vi "4155C Transfer v2.0.vi"(0 "VISA resource name in":refnum<visa-resource-name>="GPIB0::14::INSTR", 1 "Source/Common":u32(ring) items=["SMU1  ", "SMU2  ", "SMU3  ", "SMU4  ", "SMU5  ", "SMU6  "], 2 "Gate":T5={"Gate Start"=0.0, "Gate Stop"=2.0, "Gate Step (linear only)"=1.0, "Gate Compliance"=0.0001, "Gate PComp"=0.0, "Range mode"=0, "Range"=6} {"Range" max=11 scale=0.0..11.0; "Range mode" items=["Auto", "Limited", "Fixed"]; "Gate PComp" min=0.0 max=2.0 format="%^.2e"; "Gate Compliance" min=0.0 max=0.1 format="%^.2e"; "Gate Step (linear only)" min=-100.0 max=100.0 format="%^.4e"; "Gate Stop" min=-100.0 max=100.0 format="%^.4e"; "Gate Start" min=-100.0 max=100.0 format="%^.4e"}, 3 "Drain":T6={"Drain Start"=0.0, "Drain Stop"=2.0, "Drain Compliance"=0.0001, "Drain Step"=1.0, "Drain PComp"=0.0, "Range mode"=0, "Range"=6} {"Range" max=11 scale=0.0..11.0; "Range mode" items=["Auto", "Limited", "Fixed"]; "Drain PComp" min=0.0 max=2.0 format="%^.2e"; "Drain Step" min=-100.0 max=100.0 format="%^.4e"; "Drain Compliance" min=0.0 max=0.1 format="%^.2e"; "Drain Stop" min=-100.0 max=100.0 format="%^.4e"; "Drain Start" min=-100.0 max=100.0 format="%^.4e"}, 4 "Drain":u32(ring)=1 items=["SMU1  ", "SMU2  ", "SMU3  ", "SMU4  ", "SMU5  ", "SMU6  "], 5 "Timings":T4={"integration time"=0, "Short/Long integration time"=0.00064, "hold time (sec)"=0.0, "delay time (sec)"=0.0, "Step Time (0 disables)"=0.0, "sweep method"=0, "Pulse period"=0.005, "Base voltage"=0.0, "Pulse width"=0.0005} {"Pulse width" min=0.0005 max=0.1 step=0.0001 format="%.4f"; "Base voltage" min=-100.0 max=100.0 format="%^.4e"; "Pulse period" min=0.005 max=1.0 step=0.0001 format="%.4f"; "sweep method" items=["Continuous", "Pulsed"]; "Step Time (0 disables)" min=0.0 format="%.2f"; "delay time (sec)" min=0.0 format="%.4f"; "hold time (sec)" min=0.0 format="%.4f"; "Short/Long integration time" min=0.0 format="%^.0e"; "integration time" scale=0.0..2.0}, 6 "error in (no error)":errorcluster, 7 "Probe 4":cluster{"on/off":bool, "Voltage":dbl} {"Voltage" min=-100.0 max=100.0 format="%.2f"}, 8 "Gate":u32(ring)=2 items=["SMU1  ", "SMU2  ", "SMU3  ", "SMU4  ", "SMU5  ", "SMU6  "], 9 "Probe 4":u32(ring)=3 items=["SMU1  ", "SMU2  ", "SMU3  ", "SMU4  ", "SMU5  ", "SMU6  "], 10 "sweep mode":u16(ring) items=["Single", "Double"], 12 "Panel Controls":T3={"Emergency Stop"=refnum, "TransGraph Max"=1e-05, "Text/Graph (text=false)"=FALSE, "TransGraph Min"=1e-11} {"TransGraph Min" format="%.2e"; "TransGraph Max" format="%.2e"}, 13 "Standby":T1) -> (16 "VG":dbl[](array[numeric]) format="%.2f", 17 "Outparams":T2={"V2 Start"=0.0, "V2 Step"=0.0, "Number of points"=1} {"V2 Step" format="%.2f"; "V2 Start" format="%^.4e"}, 20 "VISA Resource Name out":refnum<visa-resource-name>, 22 "IS":dbl[](array[numeric]) format="%.2f", 23 "ID":dbl[](array[numeric]) format="%.2f", 25 "IG":dbl[](array[numeric]) format="%.2f", 26 "error out":errorcluster, 27 "Probe 4":dbl[](array[numeric]) format="%.2f")   [LabVIEW 2016]
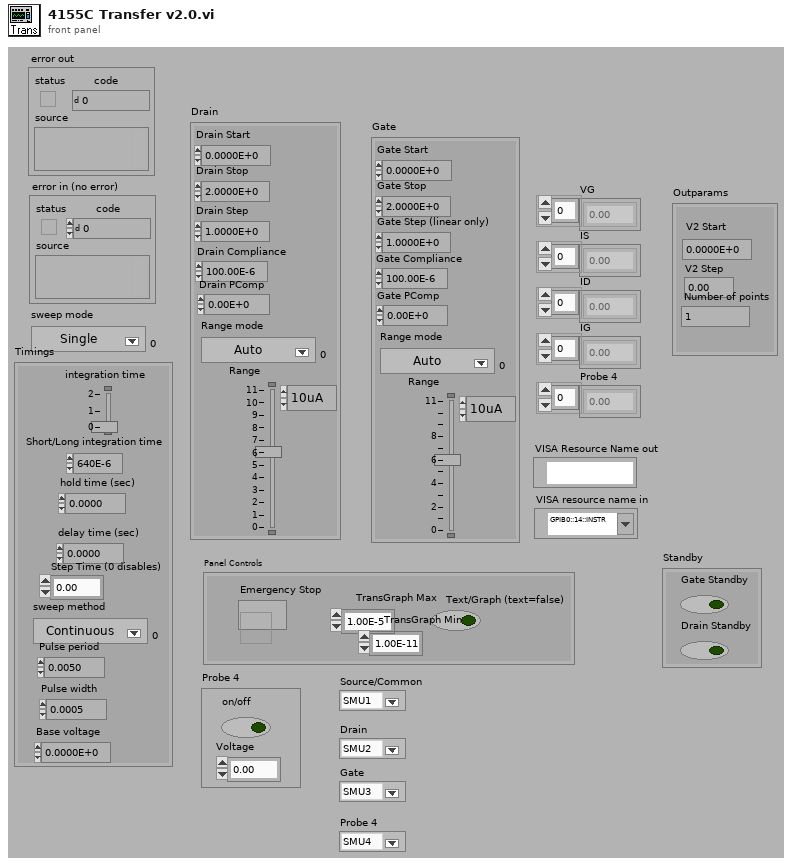
[diagram p1: front panel]
types:
  T1 = cluster{"Gate Standby":bool, "Drain Standby":bool}
  T2 = cluster{"V2 Start":dbl, "V2 Step":dbl, "Number of points":i32}
  T3 = cluster{"Emergency Stop":refnum<vi>, "TransGraph Max":dbl, "Text/Graph (text=false)":bool, "TransGraph Min":dbl}
  T4 = cluster{"integration time":u32, "Short/Long integration time":dbl, "hold time (sec)":dbl, "delay time (sec)":dbl, "Step Time (0 disables)":dbl, "sweep method":u16, "Pulse period":dbl, "Base voltage":dbl, "Pulse width":dbl}
  T5 = cluster{"Gate Start":dbl, "Gate Stop":dbl, "Gate Step (linear only)":dbl, "Gate Compliance":dbl, "Gate PComp":dbl, "Range mode":u16, "Range":u8}
  T6 = cluster{"Drain Start":dbl, "Drain Stop":dbl, "Drain Compliance":dbl, "Drain Step":dbl, "Drain PComp":dbl, "Range mode":u16, "Range":u8}
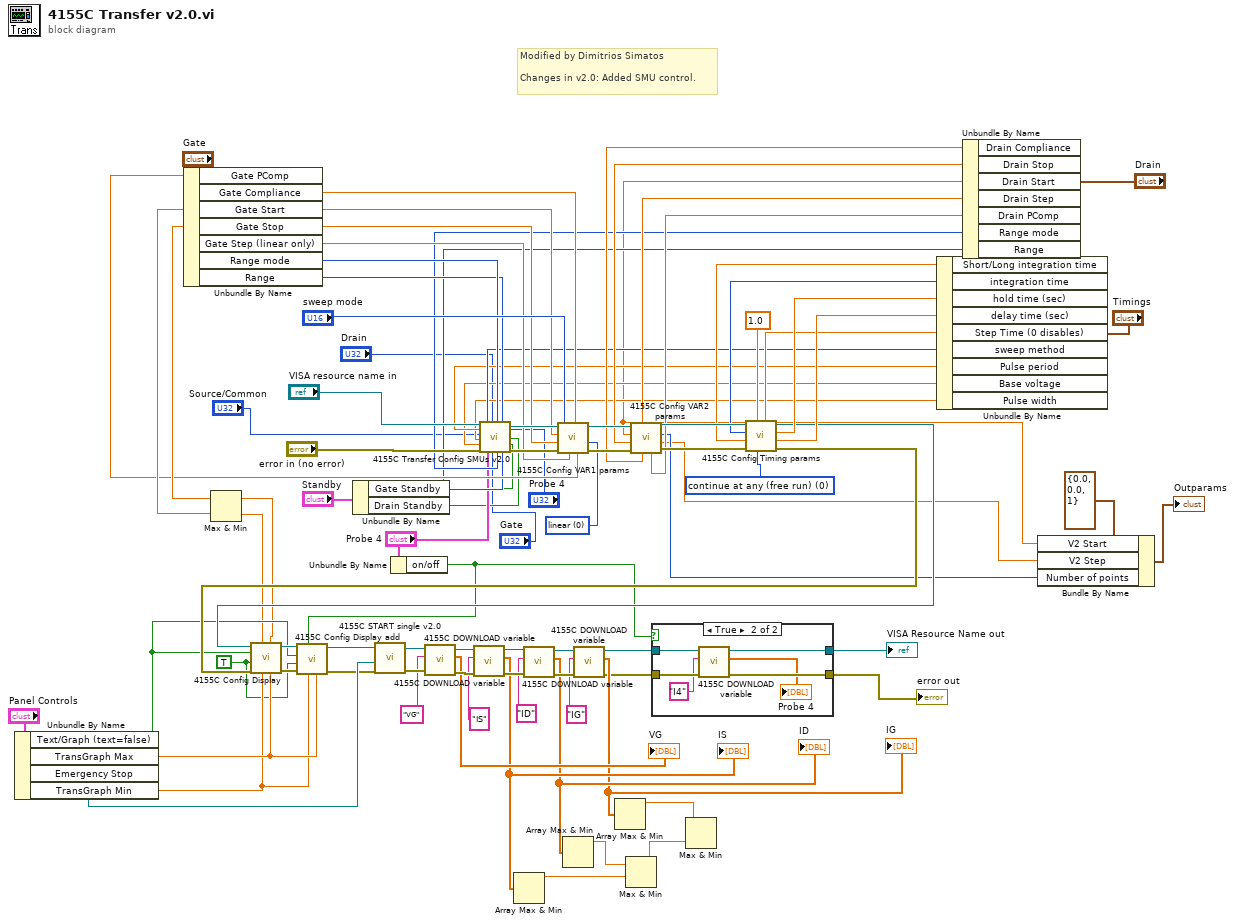
[diagram p0: block diagram]
diagram:
  w9 = TRUE ("Logarithmic")
  w73 = u8 0 items=["continue at any (free run)", "stop at any abnorm", "stop at compliance"] ("stop condition (free run:0)")
  w70 = u16 0 items=["linear", "log 10", "log 25", "log 50"] ("sweep spacing (linear: 0)")
  # "Modified by Dimitrios Simatos\n\nChanges in v2.0: Added SMU control."
  n1 = Unbundle By Name("Panel Controls") -> ("Text/Graph (text=false)"=w8:bool, "TransGraph Max"=w11:dbl, "Emergency Stop"=w40:refnum<vi>, "TransGraph Min"=w10:dbl)
  n2 = Unbundle By Name("Gate") -> ("Gate PComp"=w38:dbl, "Gate Compliance"=w59:dbl, "Gate Start"=w42:dbl, "Gate Stop"=w41:dbl, "Gate Step (linear only)"=w58:dbl, "Range mode"=w36:u16, "Range"=w35:u8)
  n3 = Max & Min(x=w41, y=w42) -> (max(x,y)=w5:dbl, min(x,y)=w6:dbl)
  n4 = Unbundle By Name("Standby") -> ("Gate Standby"=w17:bool, "Drain Standby"=w16:bool)
  n5 = Unbundle By Name("Probe 4") -> ("on/off"=w7:bool)
  n6 = Unbundle By Name("Timings") -> ("Short/Long integration time"=w75:dbl, "integration time"=w53:u32, "hold time (sec)"=w54:dbl, "delay time (sec)"=w55:dbl, "Step Time (0 disables)"=w52:dbl, "sweep method"=w32:u16, "Pulse period"=w31:dbl, "Base voltage"=w29:dbl, "Pulse width"=w30:dbl)
  n7 = Unbundle By Name("Drain") -> ("Drain Compliance"=w62:dbl, "Drain Stop"=w61:dbl, "Drain Start"=w24:dbl, "Drain Step"=w60:dbl, "Drain PComp"=w37:dbl, "Range mode"=w34:u16, "Range"=w33:u8)
  n8 = call "4155C Transfer Config SMUs v2.0.vi"("VISA resource name in"="VISA resource name in", "Pulse period"=w31, "Source/Common"="Source/Common", "Pulse width"=w30, "Base voltage"=w29, "error in (no error)"="error in (no error)", "sweep method"=w32, 7:"Probe 4"="Probe 4", "Drain"="Drain", "Gate"="Gate", "Gate mode"=w36, "Source/drain mode"=w34, "Gate Range"=w35, "Source/drain Range"=w33, 15:"Probe 4"="Probe 4", "Drain Standby"=w16, "Gate Standby"=w17) -> ("VISA Resource Name out"=w68:refnum<visa-resource-name>, "error out"=w67:errorcluster)  [unwired: 1 in]
  n9 = call "4155C Config VAR1 params.vi"("sweep spacing (linear: 0)"=w70, "power compliance (0 = OFF)"=w38, "compliance"=w59, "step (linear only)"=w58, "sweep mode"="sweep mode", "error in (no error)"=w67, "stop"=w41, "start"=w42, "VISA session"=w68) -> ("error out"=w71:errorcluster, "dup VISA resource name"=w72:refnum<visa-resource-name>)  [unwired: 1 out]
  n10 = call "4155C Config VAR2 params.vi"("power compliance (0 = OFF)"=w37, "compliance"=w62, "step"=w60, "error in (no error)"=w71, "stop"=w61, "start"=w24, "VISA session"=w72) -> ("error out"=w76:errorcluster, "Corrected Step"=w25:dbl, "Number of points"=w26:i32, "dup VISA resource name"=w77:refnum<visa-resource-name>)  [unwired: 1 in]
  n11 = call "4155C Config Timing params.vi"("delay time (sec)"=w55, "hold time (sec)"=w54, "Step Time (0 disables)"=w52, "stop condition (free run:0)"=w73, "wait time parameter"=1.0, "error in (no error)"=w76, "Short/Long integration time"=w75, "integration time"=w53, "VISA session"=w77) -> ("error out"=w44:errorcluster, "dup VISA resource name"=w43:refnum<visa-resource-name>)  [unwired: 1 in]
  n12 = call "4155C Config Display.vi"("Ymax"=w11, "Var1 Stop"=w5, "Ymin"=w10, "Var1 Start"=w6, "error in (no error)"=w44, "Logarithmic"=w9, "SPA Display"=w8, "VISA session"=w43) -> ("error out"=w12:errorcluster, "dup VISA resource name"=w15:refnum<visa-resource-name>)  [unwired: 2 in]
  n13 = call "4155C Config Display add.vi"("Ymax"=w11, "Ymin"=w10, "SMU4"=w7, "error in (no error)"=w12, "Logarithmic"=w9, "SPA Display"=w8, "VISA session"=w15) -> ("error out"=w13:errorcluster, "dup VISA resource name"=w14:refnum<visa-resource-name>)  [unwired: 3 in]
  n14 = call "4155C START single v2.0.vi"("error in (no error)"=w13, "Emergency Stop"=w40, "VISA resource name in"=w14) -> ("error out"=w88:errorcluster, "VISA Resource Name out"=w89:refnum<visa-resource-name>)  [unwired: 3 in]
  n15 = call "4155C DOWNLOAD variable.vi"("error in (no error)"=w88, "Variable name"="VG", "VISA resource name in"=w89) -> ("error out"=w86:errorcluster, "Output data"=→"VG":dbl[], "VISA Resource Name out"=w85:refnum<visa-resource-name>)  [unwired: 2 in]
  n16 = call "4155C DOWNLOAD variable.vi"("error in (no error)"=w86, "Variable name"="IS", "VISA resource name in"=w85) -> ("error out"=w82:errorcluster, "Output data"=w51:dbl[], "VISA Resource Name out"=w83:refnum<visa-resource-name>)  [unwired: 2 in]
  "IS" <- w51
  n17 = Array Max & Min(array=w51) -> (max value=w48:dbl)  [unwired: 3 out]
  n18 = call "4155C DOWNLOAD variable.vi"("error in (no error)"=w82, "Variable name"="ID", "VISA resource name in"=w83) -> ("error out"=w81:errorcluster, "Output data"=w50:dbl[], "VISA Resource Name out"=w80:refnum<visa-resource-name>)  [unwired: 2 in]
  "ID" <- w50
  n19 = Array Max & Min(array=w50) -> (max value=w47:dbl)  [unwired: 3 out]
  n20 = call "4155C DOWNLOAD variable.vi"("error in (no error)"=w81, "Variable name"="IG", "VISA resource name in"=w80) -> ("error out"=w23:errorcluster, "Output data"=w49:dbl[], "VISA Resource Name out"=w22:refnum<visa-resource-name>)  [unwired: 2 in]
  "IG" <- w49
  n21 = Array Max & Min(array=w49) -> (max value=w46:dbl)  [unwired: 3 out]
  n22 = Max & Min(x=w47, y=w48) -> (max(x,y)=w45:dbl)  [unwired: 1 out]
  n23 = case shown="True" w7 {
    tunnel: w22 -> [w91 w97]
    tunnel: [w91 w94] -> w20
    tunnel: [w90 w95] -> w21
    tunnel: w23 -> [w90 w96]
    frame False {
    }
    frame True {
      n24 = call "4155C DOWNLOAD variable.vi"("error in (no error)"=w96, "Variable name"="I4", "VISA resource name in"=w97) -> ("error out"=w95:errorcluster, "Output data"=→"Probe 4":dbl[], "VISA Resource Name out"=w94:refnum<visa-resource-name>)  [unwired: 2 in]
    }
  }
  "error out" <- w21
  "VISA Resource Name out" <- w20
  n25 = Max & Min(x=w46, y=w45) -> ()  [unwired: 2 out]
  n26 = Bundle By Name(cluster=T2 {"V2 Start"=0.0, "V2 Step"=0.0, "Number of points"=1} ("Outparams"), "V2 Start"=w24, "V2 Step"=w25, "Number of points"=w26) -> (→"Outparams":T2)
